vi "HXG2_PIDs_No-Array.vi"(0 "Calculated Values":T3, 1 "PID Cluster":T7={"PIDon-off "={"AF PID"=FALSE, "AT PID"=FALSE, "LF PID"=FALSE, "LT PID"=FALSE}, "PID"=[], "Reset PIDs"={"AF"=FALSE, "AC"=FALSE, "AH"=FALSE, "LF"=FALSE, "LC"=FALSE, "LH"=FALSE}, "AirCool Cascade"={"PID gains"={"proportional gain (Kc)"=-1.15, "integral time (Ti, min)"=2.44, "derivative time (Td, min)"=0.0}, "output range"={"output high"=100.0, "output low"=10.0}}, "LiqHeat Cascade"={"PID gains"={"proportional gain (Kc)"=3.54, "integral time (Ti, min)"=46.25, "derivative time (Td, min)"=0.0}, "output range"={"output high"=100.0, "output low"=0.0}}} {"LiqHeat Cascade"."output range"."output low" format="%.2f"; "LiqHeat Cascade"."output range"."output high" format="%.2f"; "LiqHeat Cascade"."PID gains"."derivative time (Td, min)" format="%.3f"; "LiqHeat Cascade"."PID gains"."integral time (Ti, min)" format="%.3f"; "LiqHeat Cascade"."PID gains"."proportional gain (Kc)" format="%.3f"; "AirCool Cascade"."output range"."output low" format="%.2f"; "AirCool Cascade"."output range"."output high" format="%.2f"; "AirCool Cascade"."PID gains"."derivative time (Td, min)" format="%.3f"; "AirCool Cascade"."PID gains"."integral time (Ti, min)" format="%.3f"; "AirCool Cascade"."PID gains"."proportional gain (Kc)" format="%.3f"}, 3 "AIR-LIQ Cluster":T4 {"Liq Cluster"."Liq TEMP %" min=0.0 max=100.0 step=1.0 format="%#.1f"; "Liq Cluster"."Liq FLOW %" min=0.0 max=100.0 step=1.0 format="%#.1f"; "Liq Cluster"."TLiq °F" min=40.0 max=180.0 step=1.0 format="%#.1f"; "Liq Cluster"."Mdot lbm/hr" min=0.0 max=1000.0 step=1.0 format="%#.1f"; "Air Cluster"."Air TEMP %" min=0.0 max=100.0 step=1.0 format="%#.1f"; "Air Cluster"."Air FLOW %" min=0.0 max=100.0 step=1.0 format="%#.1f"; "Air Cluster"."Tair  °F" min=-5.0 max=100.0 step=1.0 format="%#.1f"; "Air Cluster"."CFMs" min=0.0 max=200.0 step=1.0 format="%#.1f"}, 5 "error in (no error)":errorcluster, 6 "Analog In":T2, 7 "PID Ctrls":T1, 8 "Defrost?":bool) -> (14 "PID Ctrls Out":T1, 19 "error out":errorcluster)   [LabVIEW 2012]
uses:
  Controls/HXG2_PIDctrlsOUT.ctl
  Controls/HXG2_PIDCluster.ctl
  Controls/HXG2_PIDon-off.ctl
  PID/HXG2_Horizontal PID Control.ctl
  PID/HXG2_Horizontal Reset Control.ctl
  Controls/HXG2_Aircool-Cascade.ctl
  Controls/HXG2_LiqHeat-Cascade.ctl
  Controls/HXG2_AirGly-Cluster.ctl
  Controls/UI/HXG2_UI_ControlSetAir.ctl
  Controls/UI/HXG2_UI_ControlSetGly.ctl
  Controls/HXG2_Calculated.ctl
  Controls/HXG2_AnalogIn.ctl
  Modules/EnableAirGly/HXG2enable.ctl
  Controls/UI/HXG2_NumDisplayLarge.ctl
  <vilib>/addons/control/pid/pid.llb/PID Gain Schedule (DBL).vi
  <vilib>/addons/control/pid/pid.llb/PID Control Input Filter (DBL).vi
  <vilib>/addons/control/pid/pid.llb/PID Advanced (DBL).vi
  <vilib>/addons/control/pid/NI_PID_pid.lvlib
panel:
  in  "lh ctrl effort":dbl
  in  "lc ctrl effort":dbl
  out "ANALOG.TC in 3":dbl
  out "CO1":dbl format="%.2f"
  out "Means.Air In Avg":dbl
  out "SP1":dbl
  out "SP2":dbl format="%.2f"
  # "SP1"
  # "PV1"
  # "PV2"
  # "Cascade PID2 Aircool"
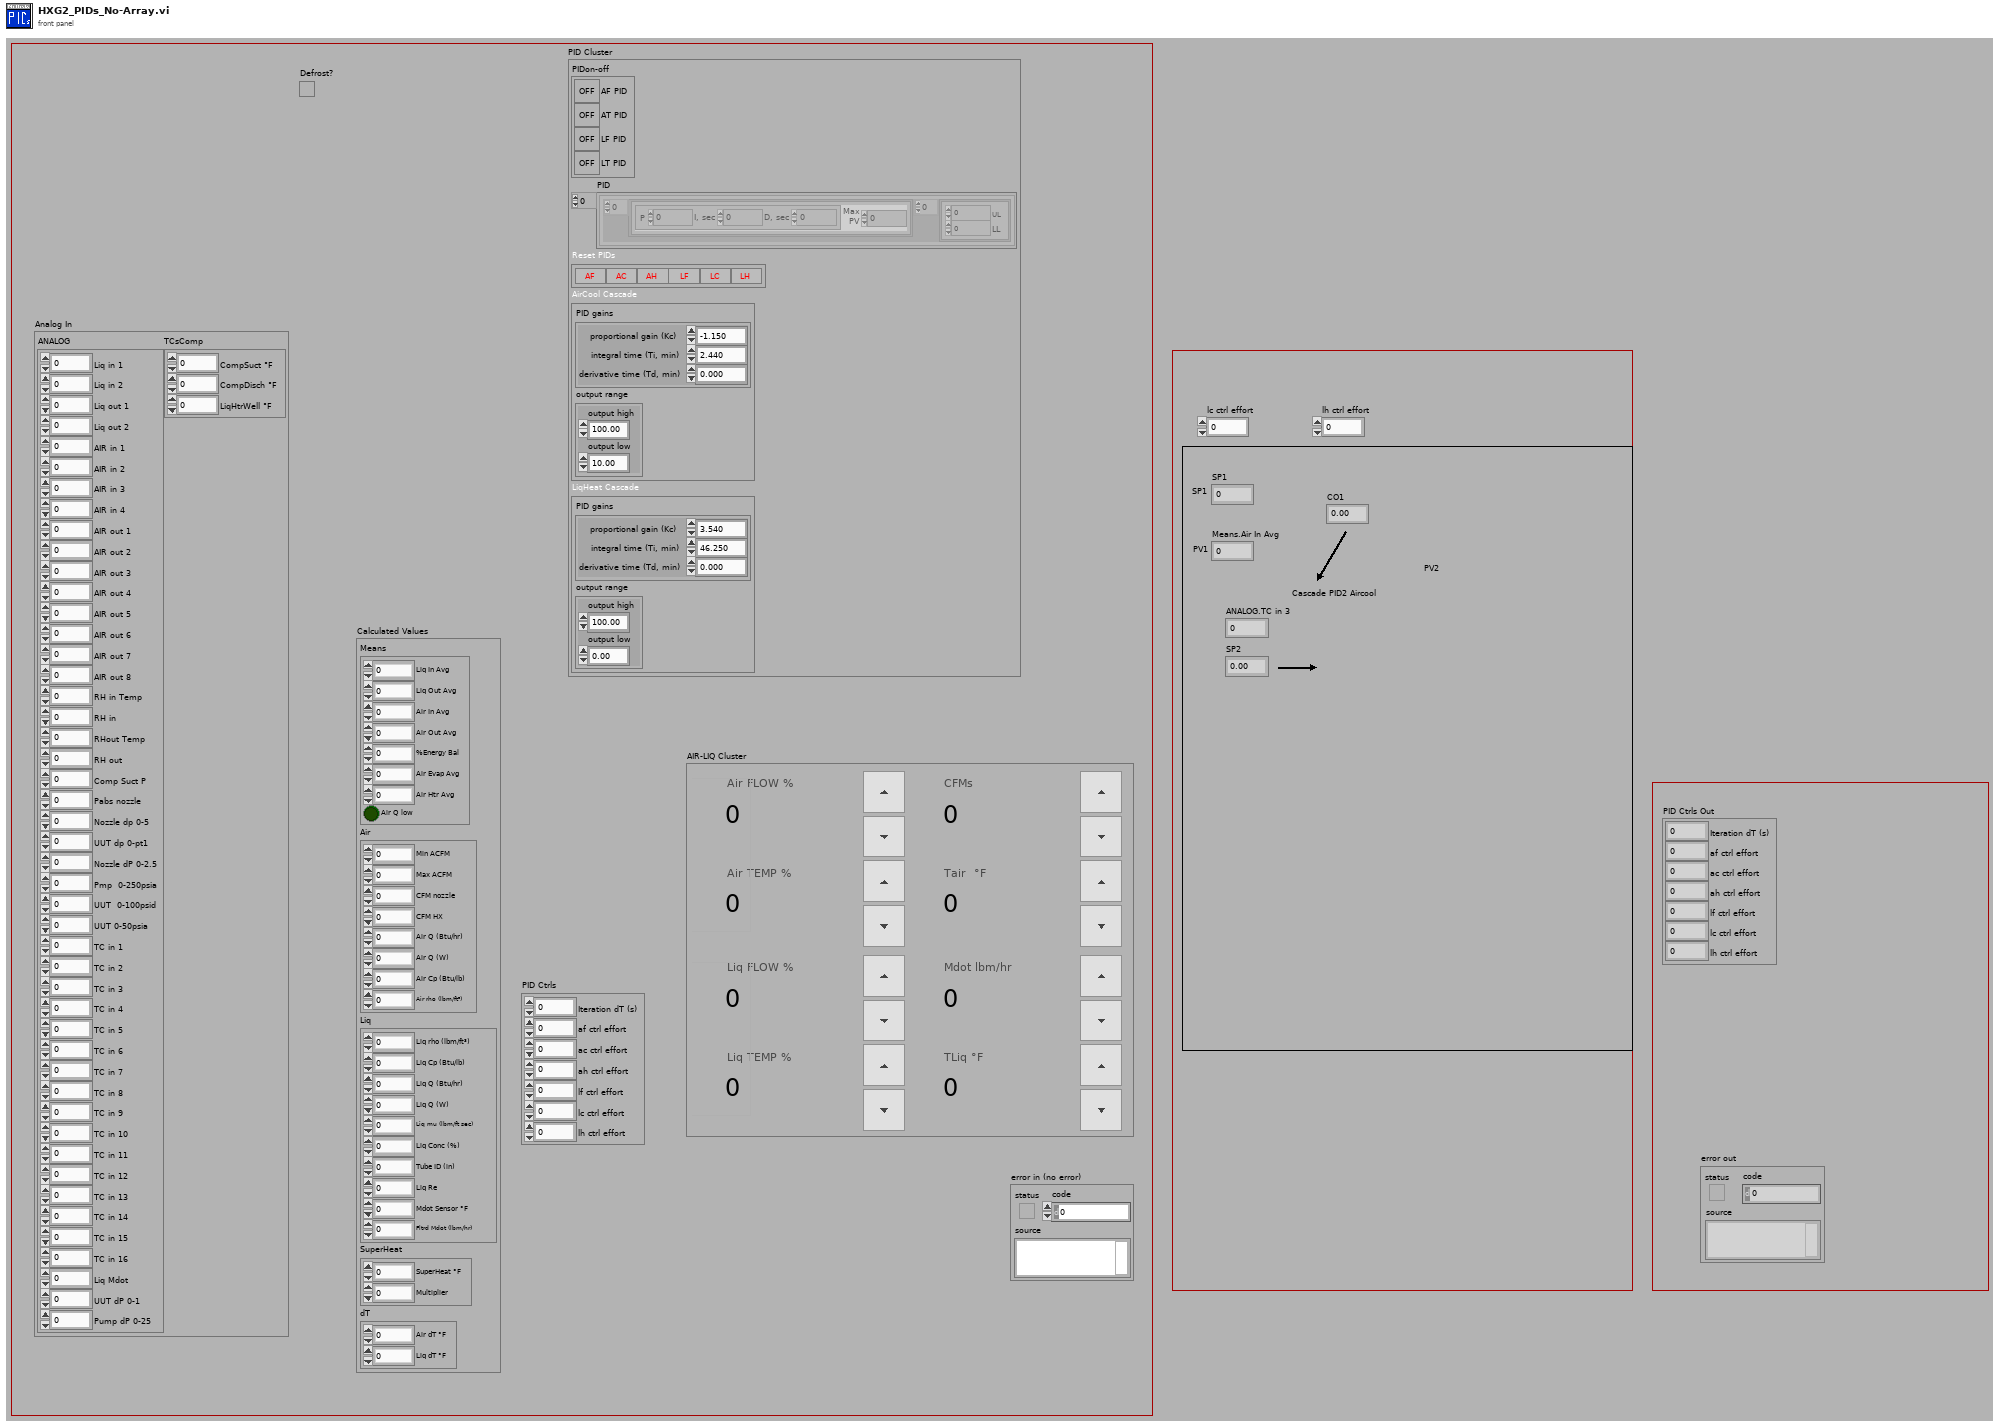
[diagram p1: front panel]
types:
  T1 = typedef "HXG2_PIDctrlsOUT.ctl" = cluster{"Iteration dT (s)":dbl, "af ctrl effort":dbl, "ac ctrl effort":dbl, "ah ctrl effort":dbl, "lf ctrl effort":dbl, "lc ctrl effort":dbl, "lh ctrl effort":dbl}
  T2 = typedef "HXG2_AnalogIn.ctl" = cluster{"ANALOG":cluster{"Liq in 1":dbl, "Liq in 2":dbl, "Liq out 1":dbl, "Liq out 2":dbl, "AIR in 1":dbl, "AIR in 2":dbl, "AIR in 3":dbl, "AIR in 4":dbl, "AIR out 1":dbl, "AIR out 2":dbl, "AIR out 3":dbl, "AIR out 4":dbl, "AIR out 5":dbl, "AIR out 6":dbl, "AIR out 7":dbl, "AIR out 8":dbl, "RH in Temp":dbl, "RH in":dbl, "RHout Temp":dbl, "RH out":dbl, "Comp Suct P":dbl, "Pabs nozzle":dbl, "Nozzle dp 0-5":dbl, "UUT dp 0-pt1":dbl, "Nozzle dP 0-2.5":dbl, "Pmp  0-250psia":dbl, "UUT  0-100psid":dbl, "UUT 0-50psia":dbl, "TC in 1":dbl, "TC in 2":dbl, "TC in 3":dbl, "TC in 4":dbl, "TC in 5":dbl, "TC in 6":dbl, "TC in 7":dbl, "TC in 8":dbl, "TC in 9":dbl, "TC in 10":dbl, "TC in 11":dbl, "TC in 12":dbl, "TC in 13":dbl, "TC in 14":dbl, "TC in 15":dbl, "TC in 16":dbl, "Liq Mdot":dbl, "UUT dP 0-1":dbl, "Pump dP 0-25":dbl}, "TCsComp":cluster{"CompSuct °F  ":dbl, "CompDisch °F":dbl, "LiqHtrWell °F":dbl}}
  T3 = typedef "HXG2_Calculated.ctl" = cluster{"Means":cluster{"Liq In Avg":dbl, "Liq Out Avg":dbl, "Air In Avg":dbl, "Air Out Avg":dbl, "%Energy Bal":dbl, "Air Evap Avg":dbl, "Air Htr Avg":dbl, "Air Q low":bool}, "Air":cluster{"Min ACFM":dbl, "Max ACFM":dbl, "CFM nozzle":dbl, "CFM HX":dbl, "Air Q (Btu/hr)":dbl, "Air Q (W)":dbl, "Air Cp (Btu/lb)":dbl, "Air rho (lbm/ft³)":dbl}, "Liq":cluster{"Liq rho (lbm/ft³)":dbl, "Liq Cp (Btu/lb)":dbl, "Liq Q (Btu/hr)":dbl, "Liq Q (W)":dbl, "Liq mu (lbm/ft sec)":dbl, "Liq Conc (%)":dbl, "Tube ID (in)":dbl, "Liq Re":dbl, "Mdot Sensor °F":dbl, "Fltrd Mdot (lbm/hr)":dbl}, "SuperHeat":cluster{"SuperHeat °F":dbl, "Multiplier":dbl}, "dT":cluster{"Air dT °F":dbl, "Liq dT °F":dbl}}
  T4 = typedef "HXG2_AirGly-Cluster.ctl" = cluster{"Air Cluster":T5, "Liq Cluster":T6}
  T5 = typedef "HXG2_UI_ControlSetAir.ctl" = cluster{"Air FLOW %":dbl, "Air TEMP % ":dbl, "CFMs":dbl, "Tair  °F":dbl}
  T6 = typedef "HXG2_UI_ControlSetGly.ctl" = cluster{"Liq FLOW %":dbl, "Liq TEMP % ":dbl, "Mdot lbm/hr":dbl, "TLiq °F":dbl}
  T7 = typedef "HXG2_PIDCluster.ctl" = cluster{"PIDon-off ":T8, "PID":T9, "Reset PIDs":T10, "AirCool Cascade":T11, "LiqHeat Cascade":T12}
  T8 = typedef "HXG2_PIDon-off.ctl" = cluster{"AF PID":bool, "AT PID":bool, "LF PID":bool, "LT PID":bool}
  T9 = typedef "HXG2_Horizontal PID Control.ctl" = cluster{"GainsArray":cluster{"Gains 2":cluster{"P":dbl, "I, sec":dbl, "D, sec":dbl}, "Max\nPV":dbl}[], "UL-LL Array":cluster{"UL":dbl, "LL  ":dbl}[]}[]
  T10 = typedef "HXG2_Horizontal Reset Control.ctl" = cluster{"AF":bool, "AC":bool, "AH":bool, "LF":bool, "LC":bool, "LH":bool}
  T11 = typedef "HXG2_Aircool-Cascade.ctl" = cluster{"PID gains":cluster{"proportional gain (Kc)":dbl, "integral time (Ti, min)":dbl, "derivative time (Td, min)":dbl}, "output range":cluster{"output high":dbl, "output low":dbl}}
  T12 = typedef "HXG2_LiqHeat-Cascade.ctl" = cluster{"PID gains":cluster{"proportional gain (Kc)":dbl, "integral time (Ti, min)":dbl, "derivative time (Td, min)":dbl}, "output range":cluster{"output high":dbl, "output low":dbl}}
  T13 = typedef "HXG2_NumDisplayLarge.ctl" = dbl
  T14 = typedef "HXG2enable.ctl" = enum16{"Write Refs", "Write", "Pass"}
  T15 = cluster{"Air-Liq Out[0]":bool, "Air-Liq Out[1]":bool}
  T16 = cluster{"PID[0]":cluster{"GainsArray":cluster{"Gains 2":cluster{"P":dbl, "I, sec":dbl, "D, sec":dbl}, "Max\nPV":dbl}[], "UL-LL Array":cluster{"UL":dbl, "LL  ":dbl}[]}, "PID[1]":cluster{"GainsArray":cluster{"Gains 2":cluster{"P":dbl, "I, sec":dbl, "D, sec":dbl}, "Max\nPV":dbl}[], "UL-LL Array":cluster{"UL":dbl, "LL  ":dbl}[]}, "PID[2]":cluster{"GainsArray":cluster{"Gains 2":cluster{"P":dbl, "I, sec":dbl, "D, sec":dbl}, "Max\nPV":dbl}[], "UL-LL Array":cluster{"UL":dbl, "LL  ":dbl}[]}, "PID[3]":cluster{"GainsArray":cluster{"Gains 2":cluster{"P":dbl, "I, sec":dbl, "D, sec":dbl}, "Max\nPV":dbl}[], "UL-LL Array":cluster{"UL":dbl, "LL  ":dbl}[]}, "PID[4]":cluster{"GainsArray":cluster{"Gains 2":cluster{"P":dbl, "I, sec":dbl, "D, sec":dbl}, "Max\nPV":dbl}[], "UL-LL Array":cluster{"UL":dbl, "LL  ":dbl}[]}, "PID[5]":cluster{"GainsArray":cluster{"Gains 2":cluster{"P":dbl, "I, sec":dbl, "D, sec":dbl}, "Max\nPV":dbl}[], "UL-LL Array":cluster{"UL":dbl, "LL  ":dbl}[]}}
  T17 = cluster{"GainsArray":cluster{"Gains 2":cluster{"P":dbl, "I, sec":dbl, "D, sec":dbl}, "Max\nPV":dbl}[], "UL-LL Array":cluster{"UL":dbl, "LL  ":dbl}[]}
  T18 = cluster{"Gains 2":cluster{"P":dbl, "I, sec":dbl, "D, sec":dbl}, "Max\nPV":dbl}[]
  T19 = cluster{"proportional gain (Kc)":dbl, "integral time (Ti, min)":dbl, "derivative time (Td, min)":dbl}
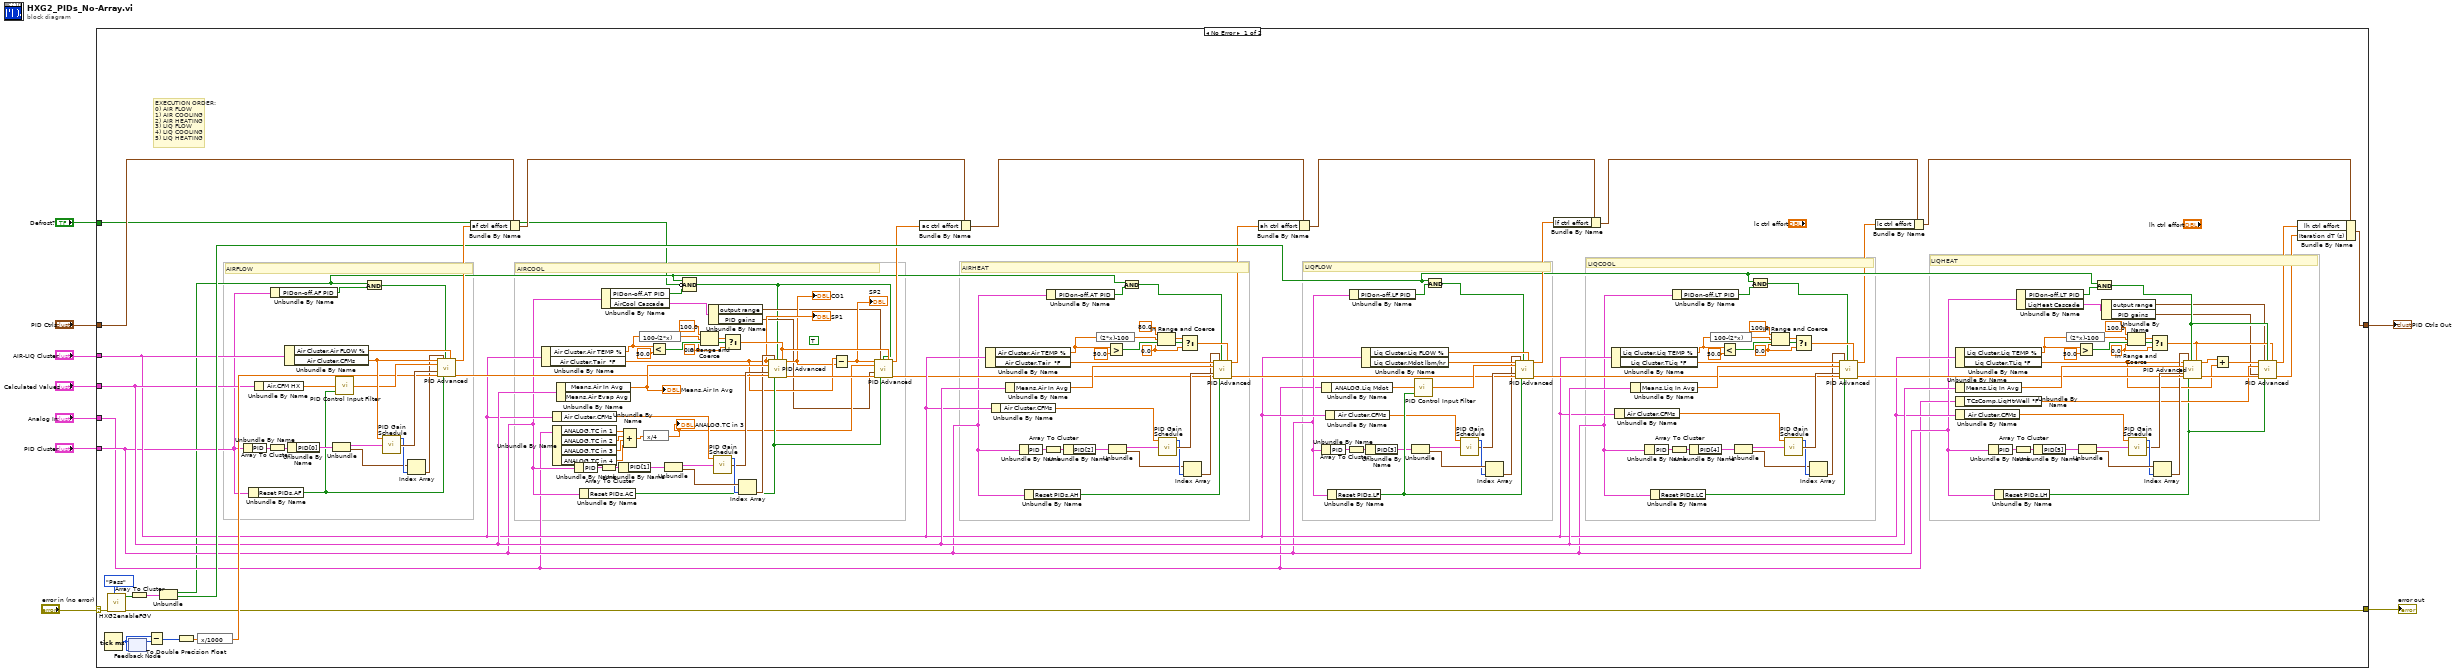
[diagram p0: block diagram]
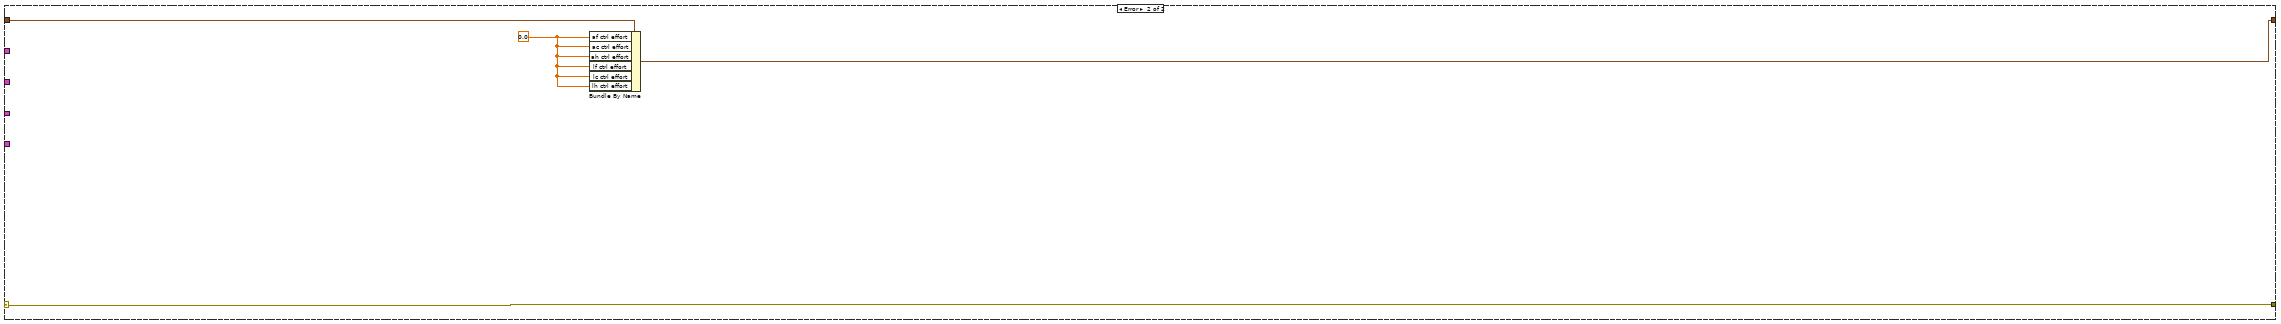
[diagram p2: hidden frame]
diagram:
  n1 = case shown="No Error" "error in (no error)" {
    selector: "error in (no error)" -> [w183 w187]
    tunnel: [w76 w187] -> w9
    tunnel: [w77 w185] -> w6
    tunnel: "PID Ctrls" -> [w168 w186]
    tunnel: "PID Cluster" -> [w24 _]
    tunnel: "AIR-LIQ Cluster" -> [w55 _]
    tunnel: "Calculated Values" -> [w63 _]
    tunnel: "Analog In" -> [w23 _]
    tunnel: "Defrost?" -> [w10 _]
    frame No Error {
      (unwired) TRUE ("coerce output to range? (T)")
      w93 = T13 0.0 ("lower limit")
      w108 = T13 0.0 ("lower limit")
      w130 = T13 0.0 ("lower limit")
      w150 = T13 0.0 ("lower limit")
      # "LIQHEAT"
      # "LIQCOOL"
      # "LIQFLOW"
      # "AIRHEAT"
      # "AIRCOOL"
      # "AIRFLOW"
      # "EXECUTION ORDER:\n0) AIR FLOW\n1) AIR COOLING\n2) AIR HEATING\n3) LIQ FLOW\n4) LIQ COOLING\n5) LIQ HEATING"
      n2 = Tick Count (ms)() -> (millisecond timer value=w180:u32)
      n3 = call "HXG2enableFGV.vi"("ENABLE Ctrl"=HXG2enable."Pass", "error in (no error)"=w183) -> ("error out"=w76:errorcluster, "Air-Liq Out"=w75:bool[])  [unwired: 7 in, 1 out]
      n4 = feedback #1(w180) -> (w178:u32)
      n5 = feedback-in #1(w180) -> ()
      n6 = Array To Cluster(array=w75) -> (cluster=w72:T15)
      n7 = Subtract(x=w180, y=w178) -> (x-y=w179:u32)
      n8 = Unbundle(w72) -> ("Air-Liq Out[0]"=w13:bool, "Air-Liq Out[1]"=w64:bool)
      n9 = To Double Precision Float(number=w179) -> (double precision float=w181:dbl)
      n10 = expression code="x/1000"(w181) -> (w155:dbl)
      n11 = Unbundle By Name(w24) -> ("PID"=w176:T9)
      n12 = Unbundle By Name(w24) -> ("Reset PIDs.AF"=w164:bool)
      n13 = Unbundle By Name(w63) -> ("Air.CFM HX"=w166:dbl)
      n14 = Array To Cluster(array=w176) -> (cluster=w175:T16)
      n15 = Unbundle By Name(w24) -> ("PIDon-off.AF PID"=w74:bool)
      n16 = Unbundle By Name(w55) -> ("Air Cluster.Air FLOW %"=w177:dbl, "Air Cluster.CFMs"=w172:dbl)
      n17 = Unbundle By Name(w175) -> ("PID[0]"=w174:T17)
      n18 = Unbundle(w174) -> ("GainsArray"=w173:T18, "UL-LL Array"=w169:cluster{"UL":dbl, "LL  ":dbl}[])
      n19 = call-poly <vilib>:"PID Control Input Filter.vi"("reinitialize? (F)"=w164, "input"=w166) -> ("output"=w165:dbl)  [unwired: 3 in]
      n20 = And(x=w13, y=w74) -> (x .and. y?=w73:bool)
      n21 = call-poly <vilib>:"PID Gain Schedule.vi"("PID gain schedule"=w173, "gain scheduling value"=w172) -> ("PID gains out"=w171:T19, "index out"=w170:i32)  [unwired: 2 in]
      n22 = Index Array(array=w169, index=w170) -> (element=w53:cluster{"UL":dbl, "LL  ":dbl})
      n23 = call-poly <vilib>:"PID Advanced.vi"("setpoint"=w172, "output range"=w53, "auto? (T)"=w73, "manual control"=w177, "process variable"=w165, "PID gains"=w171, "dt (s)"=w155, "reinitialize? (F)"=w164) -> ("output"=w167:dbl, "dt out (s)"=w154:dbl)  [unwired: 6 in]
      n24 = Bundle By Name(cluster=w168, "af ctrl effort"=w167) -> (w153:T1)
      n25 = Unbundle By Name(w55) -> ("Air Cluster.Air TEMP %"=w146:dbl, "Air Cluster.Tair  °F"=w41:dbl)
      "SP1" <- w41
      n26 = Unbundle By Name(w55) -> ("Air Cluster.CFMs"=w62:dbl)
      n27 = Unbundle By Name(w23) -> ("ANALOG.TC in 1"=w38:dbl, "ANALOG.TC in 2"=w37:dbl, "ANALOG.TC in 3"=w36:dbl, "ANALOG.TC in 4"=w16:dbl)
      n28 = Unbundle By Name(w63) -> ("Means.Air In Avg"=w163:dbl)  [unwired: 1 out]
      "Means.Air In Avg" <- w163
      n29 = Unbundle By Name(w24) -> ("PID"=w156:T9)
      n30 = Unbundle By Name(w24) -> ("Reset PIDs.AC"=w42:bool)
      n31 = Array To Cluster(array=w156) -> (cluster=w157:T16)
      n32 = Unbundle By Name(w24) -> ("PIDon-off.AT PID"=w12:bool, "AirCool Cascade"=w14:T11)
      n33 = Unbundle By Name(w157) -> ("PID[1]"=w158:T17)
      n34 = Compound Arithmetic op=ADD(w38, w37, w36, w16) -> (w35:dbl)
      n35 = expression code="100-(2*x)"(w146) -> (w149:dbl)
      n36 = expression code="x/4"(w35) -> (w34:dbl)
      "ANALOG.TC in 3" <- w34
      n37 = Less?(x=w146, y=T13 50.0) -> (x < y?=w151:bool)
      n38 = Unbundle(w158) -> ("GainsArray"=w159:T18, "UL-LL Array"=w162:cluster{"UL":dbl, "LL  ":dbl}[])
      n39 = Compound Arithmetic op=AND(w13, invert w10, w12) -> (w11:bool)
      n40 = In Range and Coerce(upper limit=T13 100.0, x=w149, lower limit=w150) -> (coerced(x)=w148:T13)  [unwired: 1 out]
      n41 = Unbundle By Name(w14) -> ("output range"=w33:cluster{"output high":dbl, "output low":dbl}, "PID gains"=w32:T19)
      n42 = call-poly <vilib>:"PID Gain Schedule.vi"("PID gain schedule"=w159, "gain scheduling value"=w62) -> ("PID gains out"=w160:T19, "index out"=w161:i32)  [unwired: 2 in]
      n43 = Select(t=w148, s=w151, f=w150) -> (s? t:f=w43:T13)
      n44 = Index Array(array=w162, index=w161) -> (element=w52:cluster{"UL":dbl, "LL  ":dbl})
      n45 = call-poly <vilib>:"PID Advanced.vi"("setpoint"=w41, "output range"=w52, "auto? (T)"=w11, "manual control"=w43, "process variable"=w163, "PID gains"=w160, "dt (s)"=w154, "reinitialize? (F)"=w42) -> ("output"=w39:dbl, "dt out (s)"=w45:dbl)  [unwired: 6 in]
      "CO1" <- w39
      n46 = Subtract(x=w41, y=w39) -> (x-y=w40:dbl)
      "SP2" <- w40
      n47 = call-poly <vilib>:"PID Advanced.vi"("setpoint"=w40, "output range"=w33, "auto? (T)"=w11, "manual control"=w43, "process variable"=w34, "PID gains"=w32, "dt (s)"=w45, "reinitialize? (F)"=w42) -> ("output"=w46:dbl, "dt out (s)"=w44:dbl)  [unwired: 6 in]
      n48 = Bundle By Name(cluster=w153, "ac ctrl effort"=w46) -> (w136:T1)
      n49 = Unbundle By Name(w55) -> ("Air Cluster.Air TEMP %"=w129:dbl, "Air Cluster.Tair  °F"=w60:dbl)
      n50 = Unbundle By Name(w55) -> ("Air Cluster.CFMs"=w61:dbl)
      n51 = Unbundle By Name(w63) -> ("Means.Air In Avg"=w138:dbl)
      n52 = Unbundle By Name(w24) -> ("PID"=w145:T9)
      n53 = Unbundle By Name(w24) -> ("Reset PIDs.AH"=w137:bool)
      n54 = Array To Cluster(array=w145) -> (cluster=w144:T16)
      n55 = Unbundle By Name(w24) -> ("PIDon-off.AT PID"=w71:bool)
      n56 = Unbundle By Name(w144) -> ("PID[2]"=w143:T17)
      n57 = expression code="(2*x)-100"(w129) -> (w132:dbl)
      n58 = Greater?(x=w129, y=T13 50.0) -> (0:w134:bool)
      n59 = Unbundle(w143) -> ("GainsArray"=w142:T18, "UL-LL Array"=w139:cluster{"UL":dbl, "LL  ":dbl}[])
      n60 = And(x=w13, y=w71) -> (x .and. y?=w70:bool)
      n61 = In Range and Coerce(upper limit=T13 80.0, x=w132, lower limit=w130) -> (coerced(x)=w131:T13)  [unwired: 1 out]
      n62 = call-poly <vilib>:"PID Gain Schedule.vi"("PID gain schedule"=w142, "gain scheduling value"=w61) -> ("PID gains out"=w141:T19, "index out"=w140:i32)  [unwired: 2 in]
      n63 = Select(t=w131, s=w134, f=w130) -> (s? t:f=w128:T13)
      n64 = Index Array(array=w139, index=w140) -> (element=w51:cluster{"UL":dbl, "LL  ":dbl})
      n65 = call-poly <vilib>:"PID Advanced.vi"("setpoint"=w60, "output range"=w51, "auto? (T)"=w70, "manual control"=w128, "process variable"=w138, "PID gains"=w141, "dt (s)"=w44, "reinitialize? (F)"=w137) -> ("output"=w47:dbl, "dt out (s)"=w116:dbl)  [unwired: 6 in]
      n66 = Bundle By Name(cluster=w136, "ah ctrl effort"=w47) -> (w115:T1)
      n67 = Unbundle By Name(w24) -> ("PID"=w118:T9)
      n68 = Unbundle By Name(w23) -> ("ANALOG.Liq Mdot"=w125:dbl)
      n69 = Unbundle By Name(w55) -> ("Air Cluster.CFMs"=w59:dbl)
      n70 = Unbundle By Name(w24) -> ("Reset PIDs.LF"=w127:bool)
      n71 = Array To Cluster(array=w118) -> (cluster=w119:T16)
      n72 = Unbundle By Name(w24) -> ("PIDon-off.LF PID"=w69:bool)
      n73 = Unbundle By Name(w55) -> ("Liq Cluster.Liq FLOW %"=w117:dbl, "Liq Cluster.Mdot lbm/hr"=w58:dbl)
      n74 = Unbundle By Name(w119) -> ("PID[3]"=w120:T17)
      n75 = Unbundle(w120) -> ("GainsArray"=w121:T18, "UL-LL Array"=w124:cluster{"UL":dbl, "LL  ":dbl}[])
      n76 = call-poly <vilib>:"PID Control Input Filter.vi"("reinitialize? (F)"=w127, "input"=w125) -> ("output"=w126:dbl)  [unwired: 3 in]
      n77 = And(x=w64, y=w69) -> (x .and. y?=w68:bool)
      n78 = call-poly <vilib>:"PID Gain Schedule.vi"("PID gain schedule"=w121, "gain scheduling value"=w59) -> ("PID gains out"=w122:T19, "index out"=w123:i32)  [unwired: 2 in]
      n79 = Index Array(array=w124, index=w123) -> (element=w50:cluster{"UL":dbl, "LL  ":dbl})
      n80 = call-poly <vilib>:"PID Advanced.vi"("setpoint"=w58, "output range"=w50, "auto? (T)"=w68, "manual control"=w117, "process variable"=w126, "PID gains"=w122, "dt (s)"=w116, "reinitialize? (F)"=w127) -> ("output"=w114:dbl, "dt out (s)"=w96:dbl)  [unwired: 6 in]
      n81 = Bundle By Name(cluster=w115, "lf ctrl effort"=w114) -> (w95:T1)
      n82 = Unbundle By Name(w55) -> ("Liq Cluster.Liq TEMP %"=w112:dbl, "Liq Cluster.TLiq °F"=w56:dbl)
      n83 = Unbundle By Name(w55) -> ("Air Cluster.CFMs"=w57:dbl)
      n84 = Unbundle By Name(w63) -> ("Means.Liq In Avg"=w98:dbl)
      n85 = Unbundle By Name(w24) -> ("PID"=w105:T9)
      n86 = Unbundle By Name(w24) -> ("Reset PIDs.LC"=w97:bool)
      n87 = Array To Cluster(array=w105) -> (cluster=w104:T16)
      n88 = Unbundle By Name(w24) -> ("PIDon-off.LT PID"=w67:bool)
      n89 = Unbundle By Name(w104) -> ("PID[4]"=w103:T17)
      n90 = expression code="100-(2*x)"(w112) -> (w109:dbl)
      n91 = Less?(x=w112, y=T13 50.0) -> (x < y?=w107:bool)
      n92 = Unbundle(w103) -> ("GainsArray"=w102:T18, "UL-LL Array"=w99:cluster{"UL":dbl, "LL  ":dbl}[])
      n93 = And(x=w64, y=w67) -> (x .and. y?=w66:bool)
      n94 = In Range and Coerce(upper limit=T13 100.0, x=w109, lower limit=w108) -> (coerced(x)=w110:T13)  [unwired: 1 out]
      n95 = call-poly <vilib>:"PID Gain Schedule.vi"("PID gain schedule"=w102, "gain scheduling value"=w57) -> ("PID gains out"=w101:T19, "index out"=w100:i32)  [unwired: 2 in]
      n96 = Select(t=w110, s=w107, f=w108) -> (s? t:f=w113:T13)
      n97 = Index Array(array=w99, index=w100) -> (element=w49:cluster{"UL":dbl, "LL  ":dbl})
      n98 = call-poly <vilib>:"PID Advanced.vi"("setpoint"=w56, "output range"=w49, "auto? (T)"=w66, "manual control"=w113, "process variable"=w98, "PID gains"=w101, "dt (s)"=w96, "reinitialize? (F)"=w97) -> ("output"=w18:dbl, "dt out (s)"=w79:dbl)  [unwired: 6 in]
      n99 = Bundle By Name(cluster=w95, "lc ctrl effort"=w18) -> (w78:T1)
      n100 = Unbundle By Name(w55) -> ("Liq Cluster.Liq TEMP %"=w94:dbl, "Liq Cluster.TLiq °F"=w27:dbl)
      n101 = Unbundle By Name(w63) -> ("Means.Liq In Avg"=w87:dbl)
      n102 = Unbundle By Name(w23) -> ("TCsComp.LiqHtrWell °F"=w22:dbl)
      n103 = Unbundle By Name(w55) -> ("Air Cluster.CFMs"=w54:dbl)
      n104 = Unbundle By Name(w24) -> ("PID"=w80:T9)
      n105 = Unbundle By Name(w24) -> ("Reset PIDs.LH"=w21:bool)
      n106 = Array To Cluster(array=w80) -> (cluster=w81:T16)
      n107 = Unbundle By Name(w24) -> ("PIDon-off.LT PID"=w65:bool, "LiqHeat Cascade"=w15:T12)
      n108 = Unbundle By Name(w81) -> ("PID[5]"=w82:T17)
      n109 = expression code="(2*x)-100"(w94) -> (w91:dbl)
      n110 = Greater?(x=w94, y=T13 50.0) -> (0:w89:bool)
      n111 = Unbundle(w82) -> ("GainsArray"=w83:T18, "UL-LL Array"=w86:cluster{"UL":dbl, "LL  ":dbl}[])
      n112 = And(x=w64, y=w65) -> (x .and. y?=w30:bool)
      n113 = Unbundle By Name(w15) -> ("output range"=w17:cluster{"output high":dbl, "output low":dbl}, "PID gains"=w20:T19)
      n114 = In Range and Coerce(upper limit=T13 100.0, x=w91, lower limit=w93) -> (coerced(x)=w92:T13)  [unwired: 1 out]
      n115 = call-poly <vilib>:"PID Gain Schedule.vi"("PID gain schedule"=w83, "gain scheduling value"=w54) -> ("PID gains out"=w84:T19, "index out"=w85:i32)  [unwired: 2 in]
      n116 = Select(t=w92, s=w89, f=w93) -> (s? t:f=w29:T13)
      n117 = Index Array(array=w86, index=w85) -> (element=w48:cluster{"UL":dbl, "LL  ":dbl})
      n118 = call-poly <vilib>:"PID Advanced.vi"("setpoint"=w27, "output range"=w48, "auto? (T)"=w30, "manual control"=w29, "process variable"=w87, "PID gains"=w84, "dt (s)"=w79, "reinitialize? (F)"=w21) -> ("output"=w26:dbl, "dt out (s)"=w31:dbl)  [unwired: 6 in]
      n119 = Add(x=w26, y=w27) -> (x+y=w25:dbl)
      n120 = call-poly <vilib>:"PID Advanced.vi"("setpoint"=w25, "output range"=w17, "auto? (T)"=w30, "manual control"=w29, "process variable"=w22, "PID gains"=w20, "dt (s)"=w31, "reinitialize? (F)"=w21) -> ("output"=w19:dbl, "dt out (s)"=w28:dbl)  [unwired: 6 in]
      n121 = Bundle By Name(cluster=w78, "lh ctrl effort"=w19, "Iteration dT (s)"=w28) -> (w77:T1)
    }
    frame Error {
      w184 = 0.0 ("af ctrl effort")
      n122 = Bundle By Name(cluster=w186, "af ctrl effort"=w184, "ac ctrl effort"=w184, "ah ctrl effort"=w184, "lf ctrl effort"=w184, "lc ctrl effort"=w184, "lh ctrl effort"=w184) -> (w185:T1)
    }
  }
  "error out" <- w9
  "PID Ctrls Out" <- w6
